vi "海流计全局变量.vi"() -> ()   [LabVIEW 2016, in "AADI5400.lvlib"]
uses:
  AADI5400.lvlib
panel:
  out "时间间隔":u32
  in  "波特率":u32=115200
  in  "流控制":u16(ring) items=["None", "XON/XOFF", "RTS/CTS", "XON/XOFF & RTS/CTS", "DTR/DSR", "XON/XOFF & DTR/DSR"]
  in  "海流计序列号":string
  in  "海流计型号":string
  in  "剖面海流计串口":refnum<visa-resource-name>="COM6"
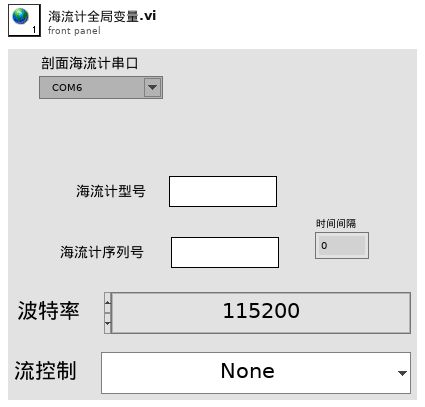
[diagram p1: front panel]
diagram:
